vi "WFGConfigure.vi"(0 "object in":refnum<class "AD2_WFG_SDK.lvclass">, 2 "WFGConfig":T1={"Running"=FALSE, "Ch1"={"idxChannel"=1, "Settings out of range"=FALSE, "Carrier"={"Frequency (Hz)"=0.0, "Amplitude (V)"=1.0, "Offset(V)"=0.0, "Symmetry(%) "=50.0, "Phase(Deg)"=0.0, "Function"=0, "Enable"=FALSE}, "Trigger"={"secRun(0=Cont)"=0.0, "secWait"=0.0, "cRepeat(0=inf)"=0, "Repeat Trigger"=FALSE, "TrigrSrc"=enum."trigrsrcNone"}, "FM Mod"={"Frequency (Hz)"=1000.0, "Amplitude (%)"=1.0, "Offset(V)"=0.0, "Symmetry(%) "=50.0, "Phase(Deg)"=0.0, "Function 2"=1, "Enable"=FALSE}}, "Ch2"={"idxChannel"=0, "Settings out of range"=FALSE, "Carrier"={"Frequency (Hz)"=1000.0, "Amplitude (V)"=1.0, "Offset(V)"=0.0, "Symmetry(%) "=50.0, "Phase(Deg)"=0.0, "Function"=1, "Enable"=FALSE}, "Trigger"={"secRun(0=Cont)"=0.0, "secWait"=0.0, "cRepeat(0=inf)"=0, "Repeat Trigger"=FALSE, "TrigrSrc"=enum."trigrsrcNone"}, "FM Mod"={"Frequency (Hz)"=1000.0, "Amplitude (%)"=1.0, "Offset(V)"=0.0, "Symmetry(%) "=50.0, "Phase(Deg)"=0.0, "Function 2"=1, "Enable"=FALSE}}, "SyncronizeState"=enum."Independent"} {"Ch2"."FM Mod"."Function 2" items=["DC"=0, "Sine"=1, "Square"=2, "Triangle"=3, "RampUp"=4, "RampDown"=5, "Noise"=6, "Pulse"=7, "Custom"=30]; "Ch2"."Carrier"."Function" items=["DC"=0, "Sine"=1, "Square"=2, "Triangle"=3, "RampUp"=4, "RampDown"=5, "Noise"=6, "Pulse"=7, "Custom"=30]; "Ch1"."FM Mod"."Function 2" items=["DC"=0, "Sine"=1, "Square"=2, "Triangle"=3, "RampUp"=4, "RampDown"=5, "Noise"=6, "Pulse"=7, "Custom"=30]; "Ch1"."Carrier"."Function" items=["DC"=0, "Sine"=1, "Square"=2, "Triangle"=3, "RampUp"=4, "RampDown"=5, "Noise"=6, "Pulse"=7, "Custom"=30]}, 5 "error in (no error)":errorcluster) -> (14 "object out":refnum<class "AD2_WFG_SDK.lvclass">, 16 "WFG config out":T1={"Running"=FALSE, "Ch1"={"idxChannel"=0, "Settings out of range"=FALSE, "Carrier"={"Frequency (Hz)"=1000.0, "Amplitude (V)"=1.0, "Offset(V)"=0.0, "Symmetry(%) "=50.0, "Phase(Deg)"=0.0, "Function"=1, "Enable"=TRUE}, "Trigger"={"secRun(0=Cont)"=0.0, "secWait"=0.0, "cRepeat(0=inf)"=0, "Repeat Trigger"=FALSE, "TrigrSrc"=enum."trigrsrcNone"}, "FM Mod"={"Frequency (Hz)"=1000.0, "Amplitude (%)"=1.0, "Offset(V)"=0.0, "Symmetry(%) "=50.0, "Phase(Deg)"=0.0, "Function 2"=1, "Enable"=FALSE}}, "Ch2"={"idxChannel"=0, "Settings out of range"=FALSE, "Carrier"={"Frequency (Hz)"=1000.0, "Amplitude (V)"=1.0, "Offset(V)"=0.0, "Symmetry(%) "=50.0, "Phase(Deg)"=0.0, "Function"=1, "Enable"=TRUE}, "Trigger"={"secRun(0=Cont)"=0.0, "secWait"=0.0, "cRepeat(0=inf)"=0, "Repeat Trigger"=FALSE, "TrigrSrc"=enum."trigrsrcNone"}, "FM Mod"={"Frequency (Hz)"=1000.0, "Amplitude (%)"=1.0, "Offset(V)"=0.0, "Symmetry(%) "=50.0, "Phase(Deg)"=0.0, "Function 2"=1, "Enable"=FALSE}}, "SyncronizeState"=enum."Independent"} {"Ch2"."FM Mod"."Function 2" items=["DC"=0, "Sine"=1, "Square"=2, "Triangle"=3, "RampUp"=4, "RampDown"=5, "Noise"=6, "Pulse"=7, "Custom"=30]; "Ch2"."Carrier"."Function" items=["DC"=0, "Sine"=1, "Square"=2, "Triangle"=3, "RampUp"=4, "RampDown"=5, "Noise"=6, "Pulse"=7, "Custom"=30]; "Ch1"."FM Mod"."Function 2" items=["DC"=0, "Sine"=1, "Square"=2, "Triangle"=3, "RampUp"=4, "RampDown"=5, "Noise"=6, "Pulse"=7, "Custom"=30]; "Ch1"."Carrier"."Function" items=["DC"=0, "Sine"=1, "Square"=2, "Triangle"=3, "RampUp"=4, "RampDown"=5, "Noise"=6, "Pulse"=7, "Custom"=30]}, 19 "error out":errorcluster)   [LabVIEW 2021, in "AD2_WFG_SDK.lvclass"]
uses:
  AD2_WFG_SDK.lvclass
  WFG.ctl
  WFGCh.ctl
  AD2TriggerSources.ctl
  AD2_SDK_class/AD2_SDK.lvclass
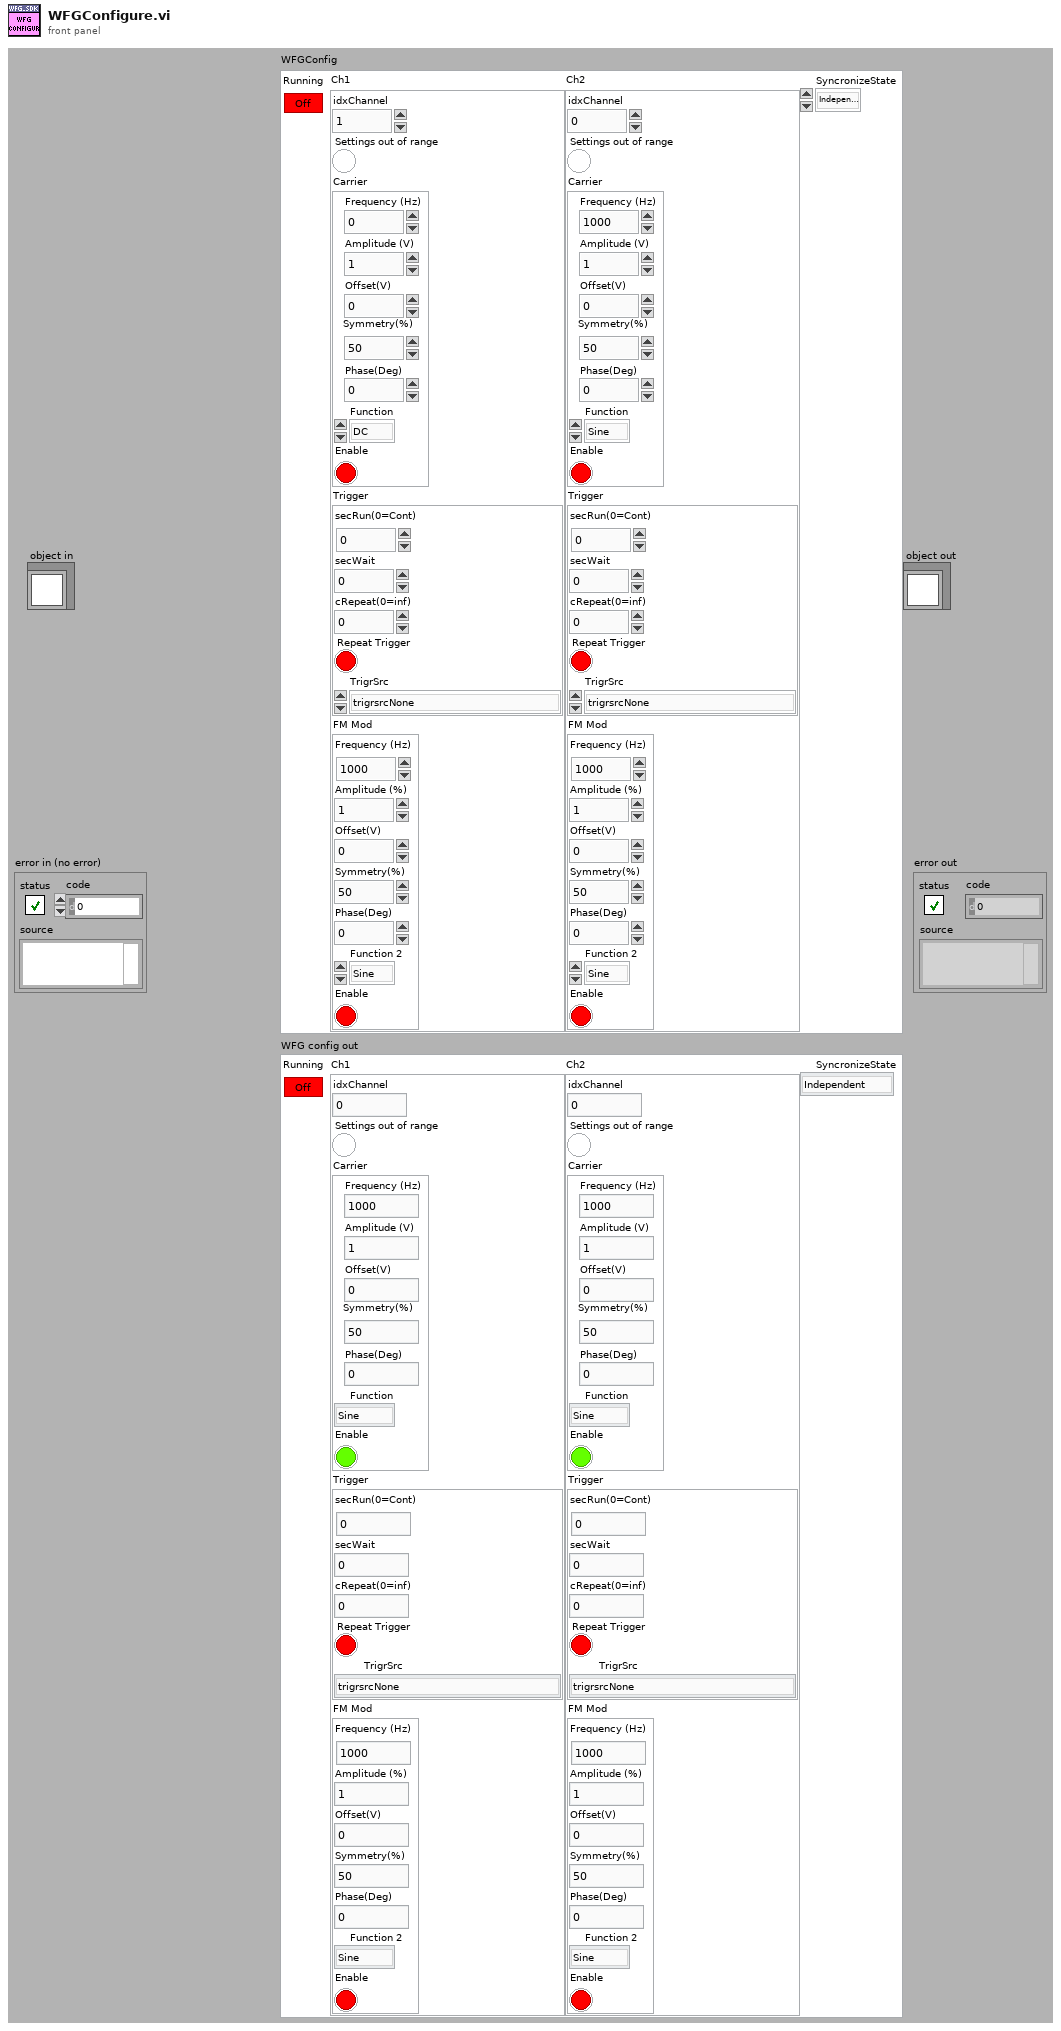
[diagram p1: front panel]
types:
  T1 = typedef "AD2_WFG_SDK.lvclass/WFG.ctl" = cluster{"Running":bool, "Ch1":T2, "Ch2":T2, "SyncronizeState":enum16{"Independent", "Ch1Master", "Ch2Master"}}
  T2 = typedef "AD2_WFG_SDK.lvclass/WFGCh.ctl" = cluster{"idxChannel":i32, "Settings out of range":bool, "Carrier":cluster{"Frequency (Hz)":dbl, "Amplitude (V)":dbl, "Offset(V)":dbl, "Symmetry(%) ":dbl, "Phase(Deg)":dbl, "Function":u16, "Enable":bool}, "Trigger":cluster{"secRun(0=Cont)":dbl, "secWait":dbl, "cRepeat(0=inf)":i32, "Repeat Trigger":bool, "TrigrSrc":T3}, "FM Mod":cluster{"Frequency (Hz)":dbl, "Amplitude (%)":dbl, "Offset(V)":dbl, "Symmetry(%) ":dbl, "Phase(Deg)":dbl, "Function 2":u16, "Enable":bool}}
  T3 = typedef "AD2_SDK.lvclass/AD2TriggerSources.ctl" = enum8{"trigrsrcNone", "trigsrcPC", "trigsrcDetectorAnalogIn", "trigsrcDetectorDigitalIn", "trigsrcAnalogIn", "trigsrcDigitalIn", "trigsrcDigitalOut", "trigsrcAnalogOut1", "trigsrcAnalogOut2", "trigsrcAnalogOut3", "trigsrcAnalogOut4", "trigsrcExternal1", "trigsrcExternal2", "trigsrcExternal3", "trigsrcExternal4", ""}
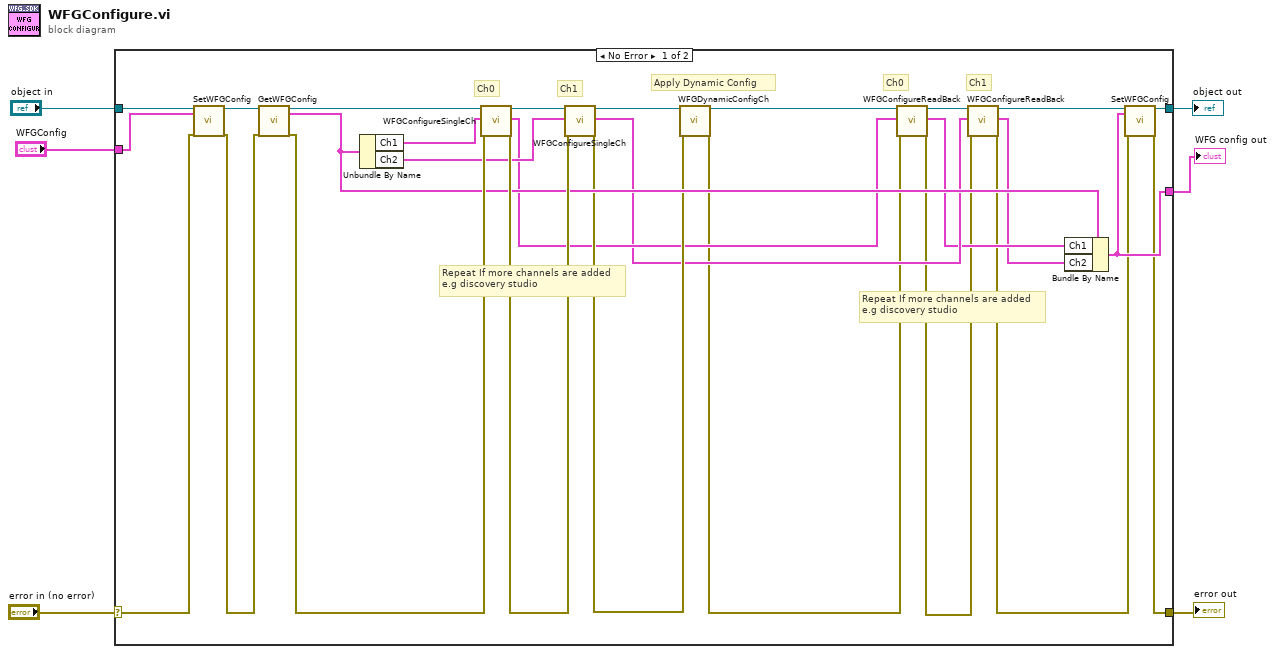
[diagram p0: block diagram]
diagram:
  n1 = case shown="No Error" "error in (no error)" {
    selector: "error in (no error)" -> [w31 w35]
    tunnel: [w7 w35] -> w5
    tunnel: [w9 w34] -> w3
    tunnel: "object in" -> [w33 w34]
    tunnel: "WFGConfig" -> [w32 _]
    tunnel: [w11 _] -> w1
    frame No Error {
      # "Repeat If more channels are added\ne.g discovery studio"
      # "Ch1"
      # "Ch0"
      # "Repeat If more channels are added\ne.g discovery studio"
      # "Apply Dynamic Config"
      # "Ch1"
      # "Ch0"
      n2 = call-dynamic "SetWFGConfig.vi"("object in"=w33, "WFG"=w32, "error in (no error)"=w31) -> ("object out"=w30:refnum<class "AD2_WFG_SDK.lvclass">, "error out"=w28:errorcluster)  [unwired: 15 in]
      n3 = call-dynamic "GetWFGConfig.vi"("object in"=w30, "error in (no error)"=w28) -> ("object out"=w29:refnum<class "AD2_WFG_SDK.lvclass">, "WFG"=w22:T1, "error out"=w27:errorcluster)  [unwired: 15 in]
      n4 = Unbundle By Name(w22) -> ("Ch1"=w26:T2, "Ch2"=w23:T2)
      n5 = call-dynamic "WFGConfigureSingleCh.vi"("object in"=w29, "Ch"=w26, "error in (no error)"=w27) -> ("object out"=w25:refnum<class "AD2_WFG_SDK.lvclass">, "Ch out"=w19:T2, "error out"=w24:errorcluster)  [unwired: 14 in]
      n6 = call-dynamic "WFGConfigureSingleCh.vi"("object in"=w25, "Ch"=w23, "error in (no error)"=w24) -> ("object out"=w21:refnum<class "AD2_WFG_SDK.lvclass">, "Ch out"=w18:T2, "error out"=w20:errorcluster)  [unwired: 14 in]
      n7 = call-dynamic "WFGDynamicConfigCh.vi"("object in"=w21, "error in (no error)"=w20) -> ("object out"=w15:refnum<class "AD2_WFG_SDK.lvclass">, "error out"=w13:errorcluster)  [unwired: 16 in]
      n8 = call-dynamic "WFGConfigureReadBack.vi"("object in"=w15, "Ch"=w19, "error in (no error)"=w13) -> ("object out"=w14:refnum<class "AD2_WFG_SDK.lvclass">, "Ch out"=w17:T2, "error out"=w12:errorcluster)  [unwired: 14 in]
      n9 = call-dynamic "WFGConfigureReadBack.vi"("object in"=w14, "Ch"=w18, "error in (no error)"=w12) -> ("object out"=w10:refnum<class "AD2_WFG_SDK.lvclass">, "Ch out"=w16:T2, "error out"=w8:errorcluster)  [unwired: 14 in]
      n10 = Bundle By Name(cluster=w22, "Ch1"=w17, "Ch2"=w16) -> (w11:T1)
      n11 = call-dynamic "SetWFGConfig.vi"("object in"=w10, "WFG"=w11, "error in (no error)"=w8) -> ("object out"=w9:refnum<class "AD2_WFG_SDK.lvclass">, "error out"=w7:errorcluster)  [unwired: 15 in]
    }
    frame Error {
    }
  }
  "error out" <- w5
  "object out" <- w3
  "WFG config out" <- w1
